vi "RGB_Force_Colour.vi"(3 "Red or Green Force":bool[][](array[boolean]), 4 "Blue":i32[][](array[numeric]), 5 "Green":i32[][](array[numeric]), 6 "Red":i32[][](array[numeric])) -> (0 "Forced Blue":i32[][](array[numeric]), 1 "Forced Green":i32[][](array[numeric]), 2 "Forced Red":i32[][](array[numeric]))   [LabVIEW 2016]
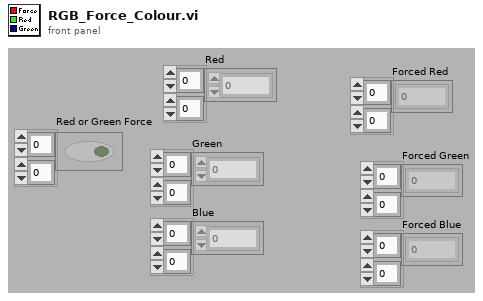
[diagram p1: front panel]
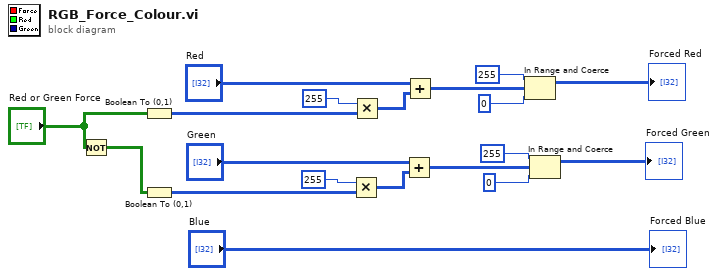
[diagram p0: block diagram]
diagram:
  n1 = Not(x="Red or Green Force") -> (.not. x?=w9:bool[][])
  n2 = Boolean To (0,1)(Boolean="Red or Green Force") -> (0, 1=w7:i16[][])
  n3 = Boolean To (0,1)(Boolean=w9) -> (0, 1=w8:i16[][])
  n4 = Multiply(x=255, y=w8) -> (x*y=w12:i32[][])
  n5 = Multiply(x=255, y=w7) -> (x*y=w15:i32[][])
  n6 = Add(x="Green", y=w12) -> (x+y=w10:i32[][])
  n7 = Add(x="Red", y=w15) -> (x+y=w13:i32[][])
  n8 = In Range and Coerce(upper limit=255, x=w13, lower limit=0) -> (coerced(x)=→"Forced Red":i32[][])  [unwired: 1 out]
  n9 = In Range and Coerce(upper limit=255, x=w10, lower limit=0) -> (coerced(x)=→"Forced Green":i32[][])  [unwired: 1 out]
  "Forced Blue" <- "Blue"
